vi "PWM to CAN.vi"(4 "s":bool, 8 "cluster manipulator 2":T3, 9 "serwa i pompa":T1={"lewy tyl "=TRUE, "prawy tyl "=TRUE, "lewy przod "=TRUE, "środek"=TRUE, "prawy przod "=TRUE, "serwo 3"=TRUE, "serwo 4 "=TRUE, "przekaznik"=TRUE}, 10 "1 bajt":u8=1, 11 "MANIPULATOR ID 3":u32) -> (1 "array of cans":T2[](array[typedef]) {"type" items=["CAN Data", "CAN Remote"]; "identifier" format="%.0x"}, 2 "druga ramka manipulator":T2 {"type" items=["CAN Data", "CAN Remote"]; "identifier" format="%.0x"}, 3 "Pierwsza ramka manipulator":T2 {"type" items=["CAN Data", "CAN Remote"]; "identifier" format="%.0x"})   [LabVIEW 2015]
uses:
  CANFrameControl.ctl
  klapki.ctl
panel:
  out "unsigned 8bit integer":u8
  out "0, 1":i16[](array[numeric])
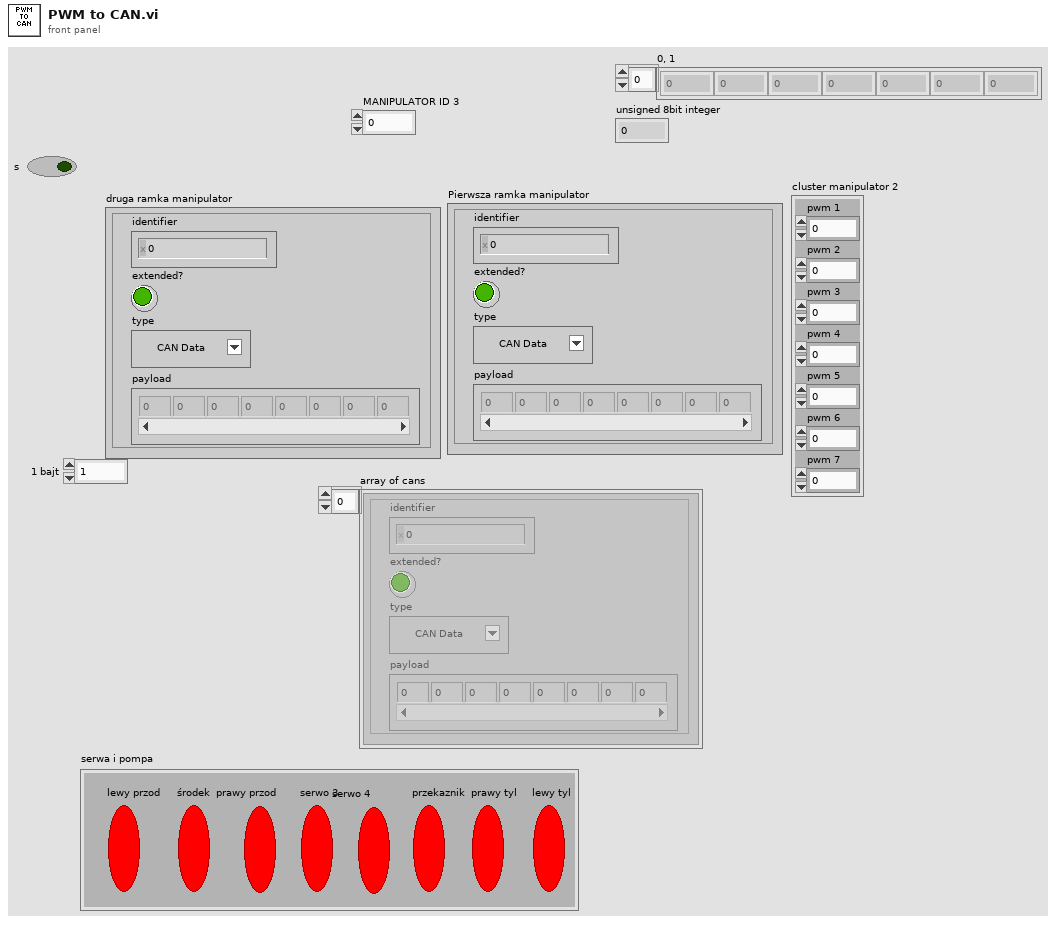
[diagram p1: front panel]
types:
  T1 = typedef "klapki.ctl" = cluster{"lewy tyl ":bool, "prawy tyl ":bool, "lewy przod ":bool, "środek":bool, "prawy przod ":bool, "serwo 3":bool, "serwo 4 ":bool, "przekaznik":bool}
  T2 = typedef "CANFrameControl.ctl" = cluster{"identifier":u32, "extended?":bool, "type":u8, "payload":u8[]}
  T3 = cluster{"pwm 1":dbl, "pwm 2":dbl, "pwm 3":dbl, "pwm 4":dbl, "pwm 5":dbl, "pwm 6":dbl, "pwm 7":dbl}
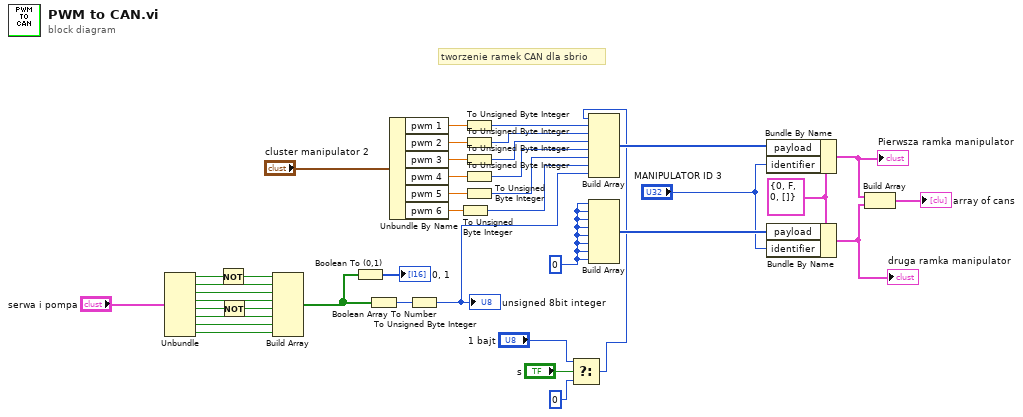
[diagram p0: block diagram]
diagram:
  w1 = u8 0
  w34 = T2 {"identifier"=0, "extended?"=FALSE, "type"=0, "payload"=[]} ("CAN frame 2")
  # "tworzenie ramek CAN dla sbrio"
  n1 = Unbundle("serwa i pompa") -> ("lewy tyl"=w7:bool, "prawy tyl"=w11:bool, "lewy przod"=w20:bool, "środek"=w19:bool, "prawy przod"=w9:bool, "serwo 3"=w15:bool, "serwo 4"=w10:bool, "przekaznik"=w14:bool)
  n2 = Not(x=w7) -> (.not. x?=w6:bool)
  n3 = Not(x=w9) -> (.not. x?=w8:bool)
  n4 = Build Array(w6, w11, w20, w19, w8, w15, w10, w14) -> (w12:bool[])
  n5 = Boolean To (0,1)(Boolean=w12) -> (0, 1=→"0, 1":i16[])
  n6 = Boolean Array To Number(Boolean array=w12) -> (number=w18:u32)
  n7 = Unbundle By Name("cluster manipulator 2") -> ("pwm 1"=w39:dbl, "pwm 2"=w38:dbl, "pwm 3"=w37:dbl, "pwm 4"=w36:dbl, "pwm 5"=w35:dbl, "pwm 6"=w28:dbl)
  n8 = To Unsigned Byte Integer(number=w18) -> (unsigned 8bit integer=w16:u8)
  "unsigned 8bit integer" <- w16
  n9 = To Unsigned Byte Integer(number=w28) -> (unsigned 8bit integer=w22:u8)
  n10 = To Unsigned Byte Integer(number=w39) -> (unsigned 8bit integer=w27:u8)
  n11 = To Unsigned Byte Integer(number=w38) -> (unsigned 8bit integer=w26:u8)
  n12 = To Unsigned Byte Integer(number=w37) -> (unsigned 8bit integer=w25:u8)
  n13 = To Unsigned Byte Integer(number=w36) -> (unsigned 8bit integer=w24:u8)
  n14 = To Unsigned Byte Integer(number=w35) -> (unsigned 8bit integer=w23:u8)
  n15 = Select(t="1 bajt", s="s", f=u8 0) -> (s? t:f=w2:u8)
  n16 = Build Array(w2, w27, w26, w25, w24, w23, w22, w16) -> (w21:u8[])
  n17 = Build Array(w1, w1, w1, w1, w1, w1, w1, w1) -> (w33:u8[])
  n18 = Bundle By Name(cluster=w34, "payload"=w21, "identifier"="MANIPULATOR ID 3") -> (w31:T2)
  "Pierwsza ramka manipulator" <- w31
  n19 = Bundle By Name(cluster=w34, "payload"=w33, "identifier"="MANIPULATOR ID 3") -> (w30:T2)
  "druga ramka manipulator" <- w30
  n20 = Build Array(w31, w30) -> (→"array of cans":T2[])
